vi "Two Axis Display.vi"(0 "Data In":T4 {"time" format="%<%.3X>T"}, 2 "Display State In":T2 {"Time_data" format="%<%.3X>T"}, 3 "Container State":T3) -> (6 "Data Out":T4 {"time" format="%<%.3X>T"}, 7 "Display State Out":T2 {"Time_data" format="%<%.3X>T"}, 8 "Action":T1)   [LabVIEW 2011, in "Two Axis.xctl"]
uses:
  Two Axis.xctl
  Two Axis Data.ctl
  <vilib>/_xctls/Container State.ctl
  Two Axis State.ctl
  <vilib>/_xctls/Action.ctl
  <vilib>/_xctls/XControlSupport.lvlib
panel:
  out "2_axis_Data":cluster{"Time_data":timestamp[], sgl[]}[](graph) caption="Vaisala Data"
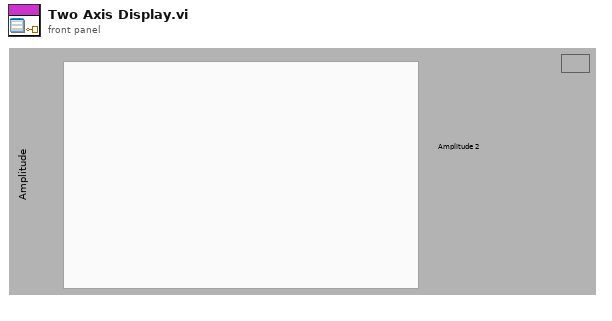
[diagram p1: front panel]
types:
  T1 = typedef "XControlSupport.lvlib/Action.ctl" = cluster{"Data Changed?":bool, "State Changed?":bool, "Action Name":string}
  T2 = typedef "Two Axis.xctl/Two Axis State.ctl" = cluster{"History":i32, "Time_data":timestamp[], "Data_Out":sgl[][], "NumPlots":i32, "LegElem":i32, "Plot Details":cluster{"Name":string, "Line Width":u8, "Line Style":u8, "Color":u32}[], "Y-Axis Labels":string[], "Title":string, "data_only?":bool}
  T3 = typedef "XControlSupport.lvlib/Container State.ctl" = cluster{"Indicator?":bool, "Run Mode?":bool, " Refnum":refnum<vi>}
  T4 = typedef "Two Axis.xctl/Two Axis Data.ctl" = cluster{"Data":sgl[], "time":timestamp}
  T5 = cluster{"Name":string, "Line Width":u8, "Line Style":u8, "Color":u32}[]
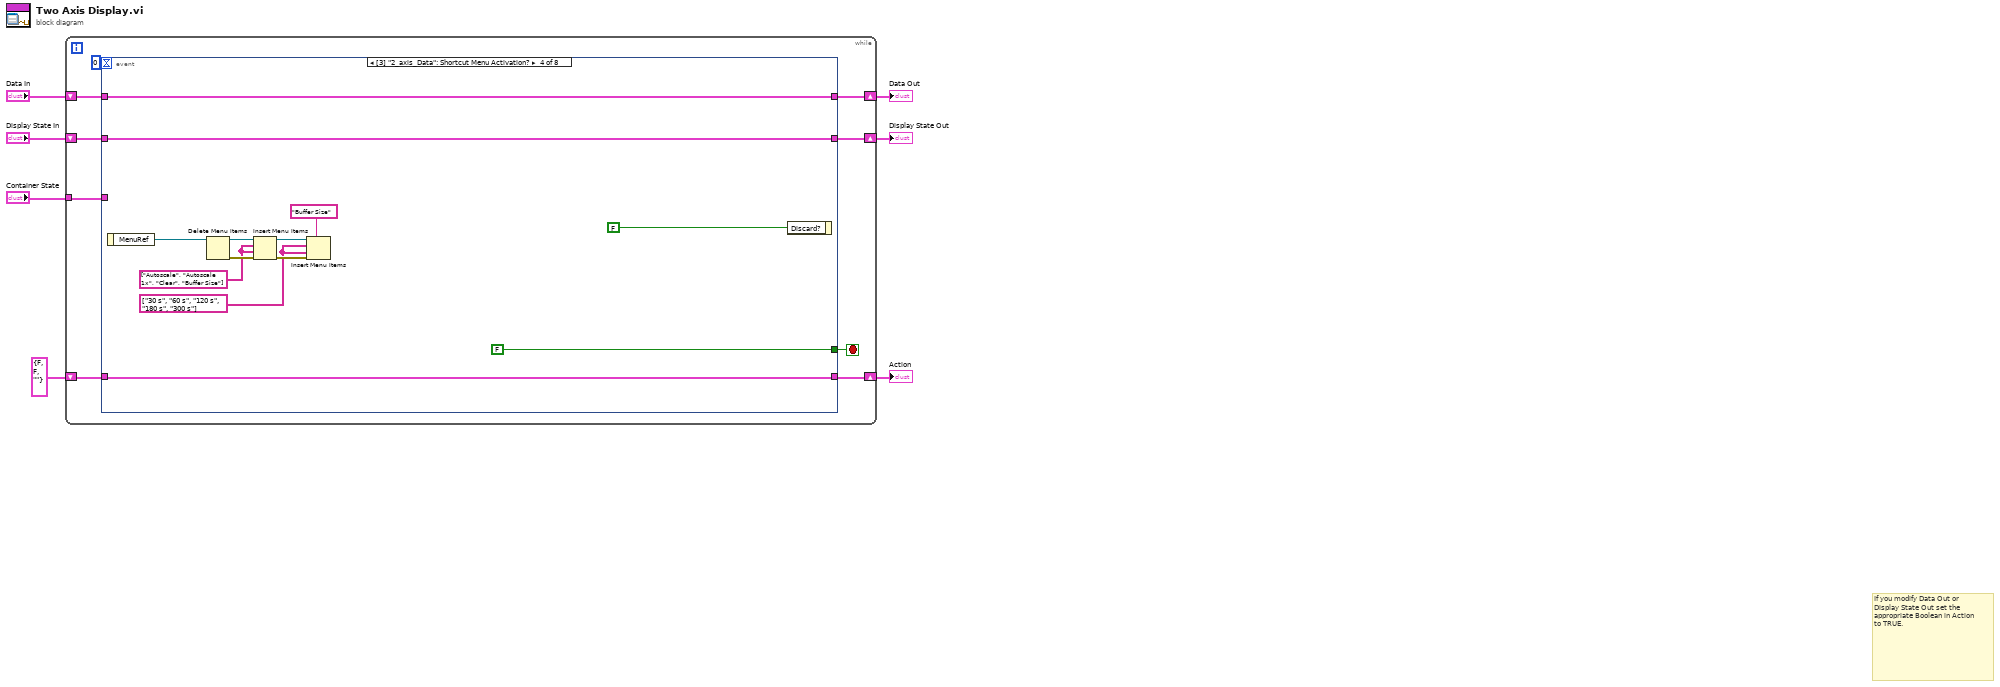
[diagram p0: block diagram]
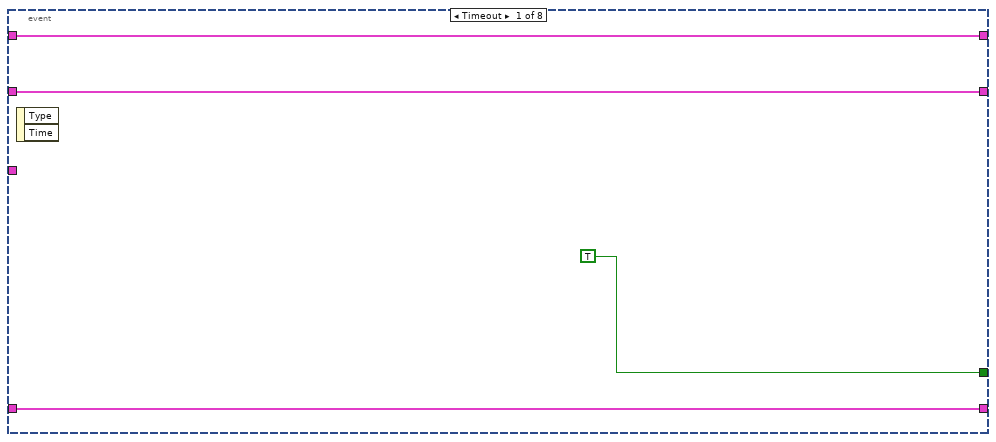
[diagram p2: hidden frame]
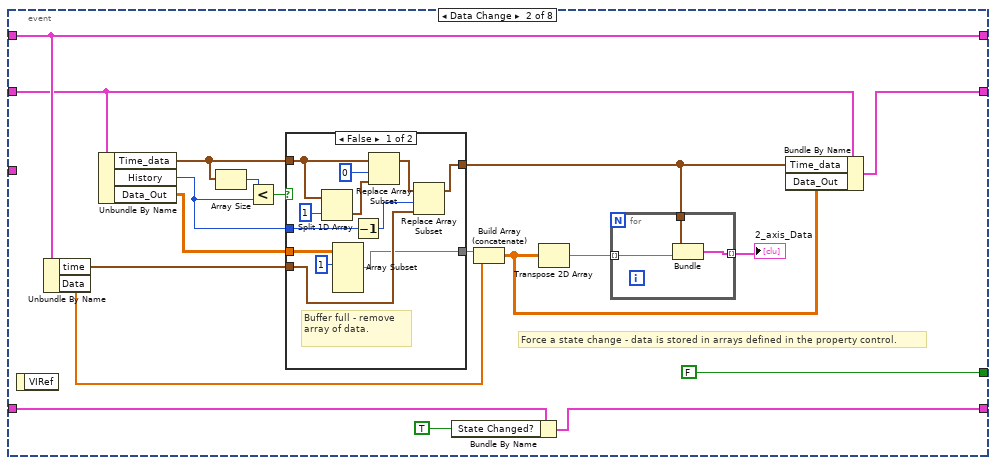
[diagram p3: hidden frame]
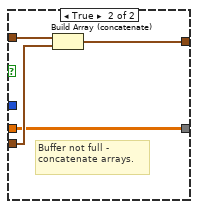
[diagram p4: hidden frame]
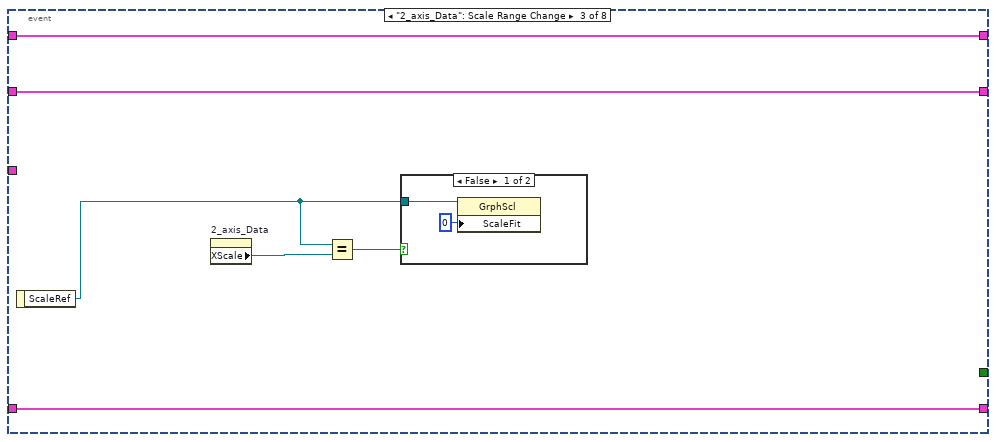
[diagram p5: hidden frame]
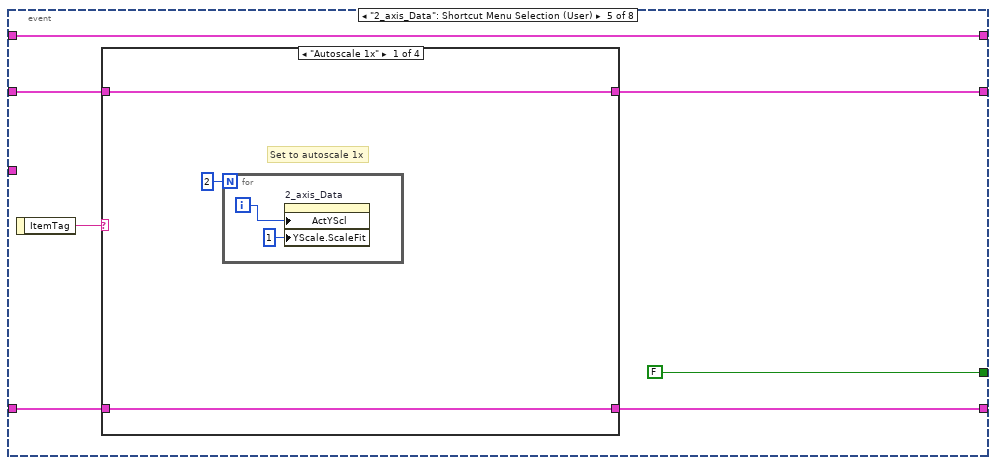
[diagram p7: hidden frame]
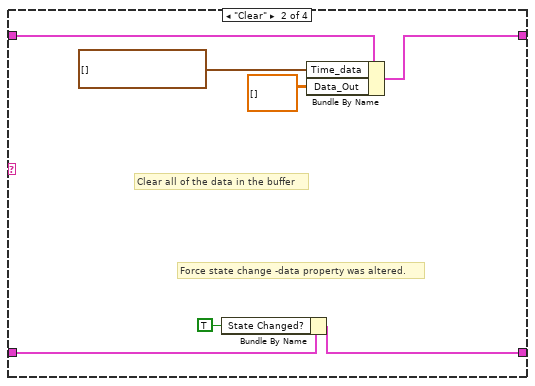
[diagram p8: hidden frame]
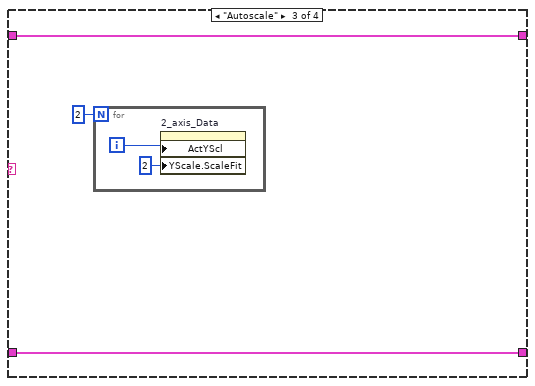
[diagram p9: hidden frame]
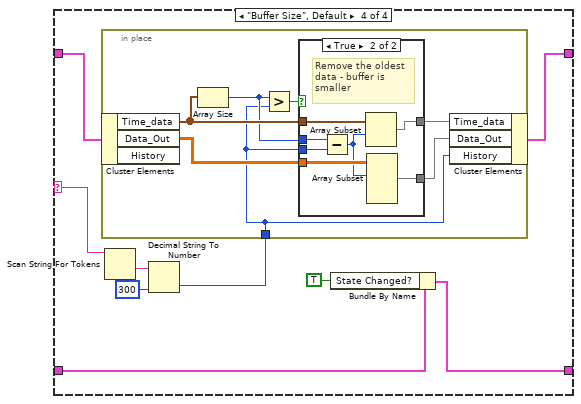
[diagram p10: hidden frame]
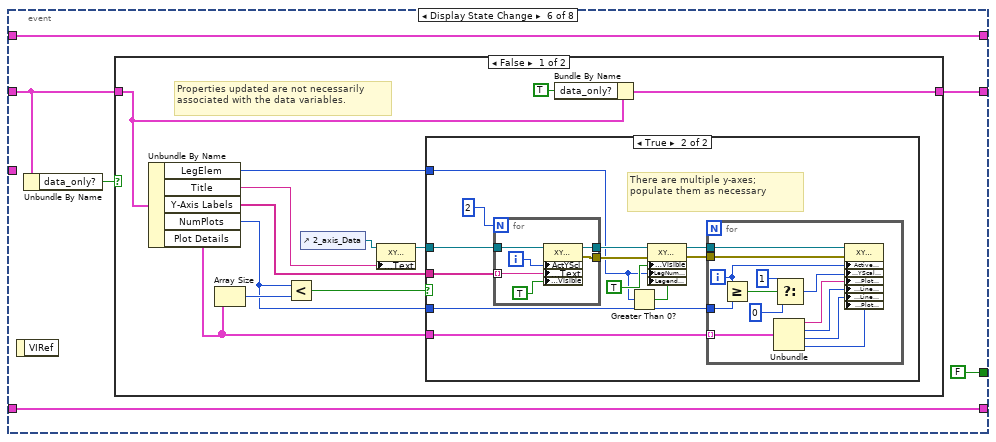
[diagram p12: hidden frame]
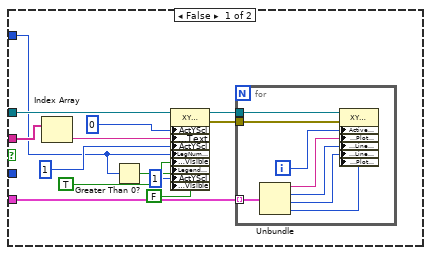
[diagram p13: hidden frame]
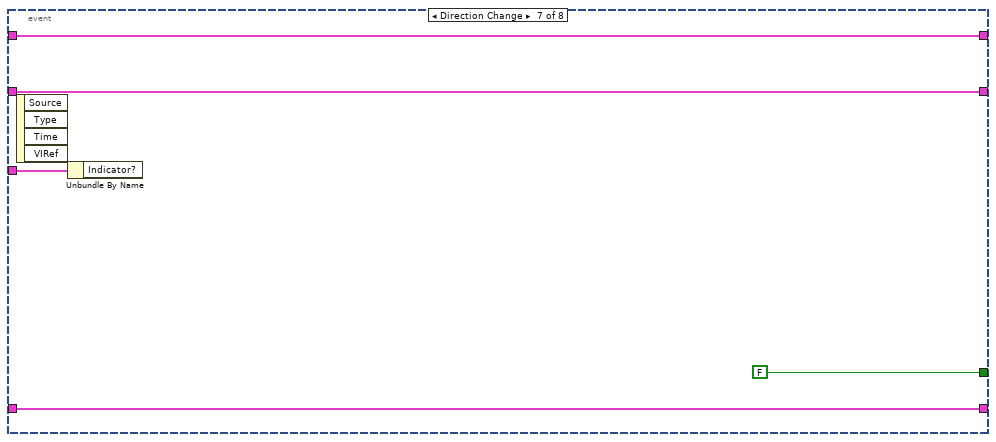
[diagram p15: hidden frame]
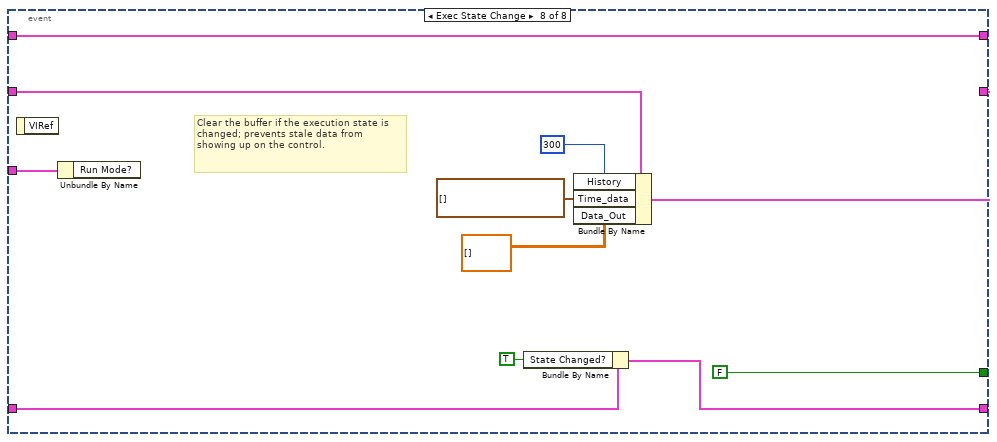
[diagram p16: hidden frame]
diagram:
  # "If you modify Data Out or\nDisplay State Out set the\nappropriate Boolean in Action\nto TRUE."
  n1 = while {
    shift-right: [w15] -> w4
    shift-left: "Display State In" -> [w16]
    tunnel: "Container State" -> [w12]
    shift-right: [w10] -> w7
    shift-left: "Data In" -> [w11]
    shift-right: [w8] -> w2
    shift-left: T1 {"Data Changed?"=FALSE, "State Changed?"=FALSE, "Action Name"=""} ("Action") -> [w9]
    stop <- w14 stop-if-true
    n2 = event shown="[3] \"2_axis_Data\": Shortcut Menu Activation?" {
      selector: _ -> [_ _ _ _ _ _ _ _]
      dyn-events: _ -> [_ _ _ _ _ _ _ _]
      timeout: 0 -> [_ _ _ _ _ _ _ _]
      tunnel: w16 -> [w18 w29 w63 w79 w84 w131 w203 w213]
      tunnel: [w18 w27 w63 w79 w82 w130 w203 w206] -> w15
      tunnel: [TRUE FALSE _ FALSE FALSE FALSE FALSE FALSE] -> w14
      tunnel: w12 -> [_ _ _ _ _ _ w204 w215]
      tunnel: w11 -> [w17 w39 w64 w78 w86 w134 w202 w214]
      tunnel: [w17 w39 w64 w78 w86 w134 w202 w214] -> w10
      tunnel: [w19 w24 w62 w77 w81 w133 w201 w207] -> w8
      tunnel: w9 -> [w19 w26 w62 w77 w83 w133 w201 w209]
      event Timeout {
        n3 = event-data() -> ()  [unwired: 1 in, 2 out]
      }
      event Data Change {
        # "Force a state change - data is stored in arrays defined in the property control."
        n4 = event-data() -> ()  [unwired: 1 in, 1 out]
        n5 = Unbundle By Name(w39) -> ("time"=w38:timestamp, "Data"=w35:sgl[])
        n6 = Unbundle By Name(w29) -> ("Time_data"=w34:timestamp[], "History"=w32:i32, "Data_Out"=w36:sgl[][])
        n7 = Array Size(array=w34) -> (size(s)=w33:i32)
        n8 = Less?(x=w33, y=w32) -> (x < y?=w31:bool)
        n9 = case shown="False" w31 {
          tunnel: w34 -> [w49 w58]
          tunnel: [w48 w56] -> w28
          tunnel: w38 -> [w47 w57]
          tunnel: w36 -> [w44 w55]
          tunnel: w32 -> [w46 _]
          tunnel: [w43 w55] -> w37
          frame False {
            # "Buffer full - remove array of data."
            n10 = Split 1D Array(array=w49, index=1) -> (second subarray=w50:timestamp[])  [unwired: 1 out]
            n11 = Array Subset(array=w44, index (row)=1 ("index")) -> (w43:sgl[][])  [unwired: 3 in]
            n12 = Decrement(x=w46) -> (x-1=w52:i32)
            n13 = Replace Array Subset(array=w49, new element=w50, index=0) -> (w53:timestamp[])
            n14 = Replace Array Subset(array=w53, new element=w47, index=w52) -> (w48:timestamp[])
          }
          frame True {
            # "Buffer not full - concatenate arrays."
            n15 = Build Array (concatenate)(w58, w57) -> (w56:timestamp[])
          }
        }
        n16 = Bundle By Name(cluster=w26, "State Changed?"=TRUE) -> (w24:T1)
        n17 = Build Array (concatenate)(w37, w35) -> (w22:sgl[][])
        n18 = Transpose 2D Array(2D array=w22) -> (transposed array=w21:sgl[][])
        n19 = for {
          tunnel: w21 -> [w40] mode=indexing
          tunnel: w28 -> [w42]
          tunnel: [w41] -> w30 mode=indexing
          n20 = Bundle("Time_data"=w42, w40) -> (w41:cluster{"Time_data":timestamp[], sgl[]})  [unwired: 1 in]
        }
        "2_axis_Data" <- w30
        n21 = Bundle By Name(cluster=w29, "Time_data"=w28, "Data_Out"=w22) -> (w27:T2)
      }
      event "2_axis_Data": Scale Range Change {
        n22 = event-data() -> ("ScaleRef"=w60:refnum<vi>)  [unwired: 1 in]
        n23 = property on="2_axis_Data" class="XYGraph (strict)"() -> ("XScale"=w61:refnum<vi>)  [unwired: 2 in, 2 out]
        n24 = Equal?(x=w60, y=w61) -> (x = y?=w59:bool)
        n25 = case shown="False" w59 {
          tunnel: w60 -> [w65 _]
          frame False {
            n26 = property class="GrphScl"(reference=w65, "ScaleFit"=u8 0 ("Scale Fit")) -> ()  [unwired: 1 in, 2 out]
          }
          frame True {
          }
        }
      }
      event "2_axis_Data": Shortcut Menu Activation? {
        w67 = string[] ["Autoscale", "Autoscale 1x", "Clear", "Buffer Size"] ("item names")
        w68 = string[] ["30 s", "60 s", "120 s", "180 s", "300 s"]
        n27 = event-data() -> ("MenuRef"=w74:refnum<k9>)  [unwired: 1 in]
        n28 = Delete Menu Items(9:w74) -> (0:w72:errorcluster, 3:w73:refnum<k9>)  [unwired: 3 in]
        n29 = Insert Menu Items(6:w72, 7:w67, 8:w67, 9:w73) -> (0:w70:errorcluster, 3:w71:refnum<k9>)  [unwired: 2 in, 1 out]
        n30 = Insert Menu Items(5:"Buffer Size", 6:w70, 7:w68, 8:w68, 9:w71) -> ()  [unwired: 1 in, 3 out]
        n31 = event-data("Discard?"=FALSE) -> ()  [unwired: 1 in, 1 out]
      }
      event "2_axis_Data": Shortcut Menu Selection (User) {
        n32 = event-data() -> ("ItemTag"=w85:string)  [unwired: 1 in]
        n33 = case shown="\"Autoscale 1x\"" w85 {
          selector: w85 -> [_ _ _ w110]
          tunnel: w84 -> [w89 w98 w101 w112]
          tunnel: w83 -> [w88 w94 w100 w106]
          tunnel: [w89 w95 w101 w111] -> w82
          tunnel: [w88 w93 w100 w104] -> w81
          frame "Autoscale 1x" {
            # "Set to autoscale 1x"
            n34 = for {
              N: 2 -> [_]
              i -> [w90]
              n35 = property on="2_axis_Data" class="XYGraph (strict)"("ActYScl"=w90, "YScale.ScaleFit"=u8 1 ("Y Scale.Scale Fit")) -> ()  [unwired: 2 in, 2 out]
            }
          }
          frame "Clear" {
            # "Force state change -data property was altered."
            # "Clear all of the data in the buffer"
            n36 = Bundle By Name(cluster=w94, "State Changed?"=TRUE) -> (w93:T1)
            n37 = Bundle By Name(cluster=w98, "Time_data"=timestamp[] [], "Data_Out"=sgl[][] []) -> (w95:T2)
          }
          frame "Autoscale" {
            n38 = for {
              N: 2 -> [_]
              i -> [w102]
              n39 = property on="2_axis_Data" class="XYGraph (strict)"("ActYScl"=w102, "YScale.ScaleFit"=u8 2 ("Y Scale.Scale Fit")) -> ()  [unwired: 2 in, 2 out]
            }
          }
          frame "Buffer Size", Default {
            n40 = Scan String For Tokens(9:w110) -> (1:w109:string)  [unwired: 5 in, 3 out]
            n41 = Decimal String To Number(string=w109, default (0L)=300 ("default (0 I32)")) -> (number=w107:i32)  [unwired: 1 in, 1 out]
            n42 = in-place {
              in-place-border: w107 -> [w113]
              n43 = in-place-cluster #1(w112) -> ("Time_data"=w118:timestamp[], "Data_Out"=w116:sgl[][])  [unwired: 1 out]
              n44 = Array Size(array=w118) -> (size(s)=w114:i32)
              n45 = Greater?(x=w114, y=w113) -> (0:w119:bool)
              n46 = case shown="True" w119 {
                tunnel: w118 -> [w121 w128]
                tunnel: [w121 w125] -> w117
                tunnel: w116 -> [w120 w124]
                tunnel: [w120 w123] -> w115
                tunnel: w114 -> [_ w127]
                tunnel: w113 -> [_ w126]
                frame False {
                  # "Buffer not filled yet or was smaller"
                }
                frame True {
                  # "Remove the oldest data - buffer is smaller"
                  n47 = Subtract(x=w127, y=w126) -> (x-y=w122:i32)
                  n48 = Array Subset(array=w128, index=w122) -> (w125:timestamp[])  [unwired: 1 in]
                  n49 = Array Subset(array=w124, index (row)=w122) -> (w123:sgl[][])  [unwired: 3 in]
                }
              }
              n50 = in-place-cluster #1("Time_data"=w117, "Data_Out"=w115, "History"=w113) -> (w111:T2)
            }
            n51 = Bundle By Name(cluster=w106, "State Changed?"=TRUE) -> (w104:T1)
          }
        }
      }
      event Display State Change {
        n52 = event-data() -> ()  [unwired: 1 in, 1 out]
        n53 = Unbundle By Name(w131) -> ("data_only?"=w132:bool)
        n54 = case shown="False" w132 {
          tunnel: w131 -> [w141 w199]
          tunnel: [w139 w199] -> w130
          frame False {
            # "Properties updated are not necessarily associated with the data variables."
            n55 = Unbundle By Name(w141) -> ("LegElem"=w142:i32, "Title"=w146:string, "Y-Axis Labels"=w135:string[], "NumPlots"=w137:i32, "Plot Details"=w136:T5)
            n56 = Array Size(array=w136) -> (size(s)=w138:i32)
            n57 = Less?(x=w137, y=w138) -> (x < y?=w144:bool)
            n58 = control-ref of="2_axis_Data"() -> (w145:refnum<vi>)
            n59 = property on="Property Node" class="XYGraph (strict)"(reference=w145, "Caption.Text"=w146) -> (reference out=w143:refnum<vi>)  [unwired: 1 in, 1 out]
            n60 = case shown="True" w144 {
              tunnel: w143 -> [w153 w178]
              tunnel: w135 -> [w158 w177]
              tunnel: w136 -> [w154 w173]
              tunnel: w137 -> [_ w172]
              tunnel: w142 -> [w150 w169]
              frame False {
                n61 = Index Array(array=w158) -> (element=w157:string)  [unwired: 1 in]
                n62 = Greater Than 0?(x=w150) -> (x > 0?=w149:bool)
                n63 = property class="XYGraph (strict)"(reference=w153, "ActYScl"=0 ("Active Y Scale"), "YScale.NameLbl.Text"=w157, "ActYScl"=1 ("Active Y Scale"), "LegNumRows"=w150, "YScale.Visible"=TRUE ("Y Scale.Visible"), "Legend Visible"=w149, "ActYScl"=1 ("Active Y Scale"), "YScale.Visible"=FALSE ("Y Scale.Visible")) -> (reference out=w155:refnum<vi>, error out=w151:errorcluster)  [unwired: 1 in]
                n64 = for {
                  tunnel: w155 -> [w167]
                  tunnel: w154 -> [w166] mode=indexing
                  tunnel: w151 -> [w160]
                  i -> [w164]
                  n65 = Unbundle(w166) -> ("Name"=w165:string, "Line Width"=w163:u8, "Line Style"=w162:u8, "Color"=w161:u32)
                  n66 = property class="XYGraph (strict)"(reference=w167, error in=w160, "Active Plot"=w164, "Plot.Plot Name"=w165, "Plot.Line Width"=w163, "Plot.Line Style"=w162, "Plot.Plot Color"=w161) -> ()  [unwired: 2 out]
                }
              }
              frame True {
                # "There are multiple y-axes; populate them as necessary"
                n67 = for {
                  N: 2 -> [_]
                  tunnel: w178 -> [w198]
                  tunnel: w177 -> [w196] mode=indexing
                  tunnel: [w195] -> w176
                  tunnel: [w193] -> w170
                  i -> [w197]
                  n68 = property class="XYGraph (strict)"(reference=w198, "ActYScl"=w197, "YScale.NameLbl.Text"=w196, "YScale.Visible"=TRUE ("Y Scale.Visible")) -> (reference out=w195:refnum<vi>, error out=w193:errorcluster)  [unwired: 1 in]
                }
                n69 = Greater Than 0?(x=w169) -> (x > 0?=w168:bool)
                n70 = property class="XYGraph (strict)"(reference=w176, error in=w170, "YScale.Visible"=TRUE ("Y Scale.Visible"), "LegNumRows"=w169, "Legend Visible"=w168) -> (reference out=w174:refnum<vi>, error out=w171:errorcluster)
                n71 = for {
                  tunnel: w174 -> [w192]
                  tunnel: w173 -> [w185] mode=indexing
                  tunnel: w172 -> [w190]
                  tunnel: w171 -> [w180]
                  i -> [w191]
                  n72 = Greater Or Equal?(x=w191, y=w190) -> (x >= y?=w189:bool)
                  n73 = Unbundle(w185) -> ("Name"=w184:string, "Line Width"=w183:u8, "Line Style"=w182:u8, "Color"=w181:u32)
                  n74 = Select(t=u32 1, s=w189, f=u32 0 ("Plot.Y Scale Index")) -> (s? t:f=w186:u32)
                  n75 = property class="XYGraph (strict)"(reference=w192, error in=w180, "Active Plot"=w191, "Plot.YScaleIdx"=w186, "Plot.Plot Name"=w184, "Plot.Line Width"=w183, "Plot.Line Style"=w182, "Plot.Plot Color"=w181) -> ()  [unwired: 2 out]
                }
              }
            }
            n76 = Bundle By Name(cluster=w141, "data_only?"=TRUE) -> (w139:T2)
          }
          frame True {
          }
        }
      }
      event Direction Change {
        n77 = event-data() -> ()  [unwired: 1 in, 4 out]
        n78 = Unbundle By Name(w204) -> ()  [unwired: 1 out]
      }
      event Exec State Change {
        # "Clear the buffer if the execution state is changed; prevents stale data from showing up on the control."
        n79 = event-data() -> ()  [unwired: 1 in, 1 out]
        n80 = Unbundle By Name(w215) -> ()  [unwired: 1 out]
        n81 = Bundle By Name(cluster=w209, "State Changed?"=TRUE) -> (w207:T1)
        n82 = Bundle By Name(cluster=w213, "History"=300, "Time_data"=timestamp[] [], "Data_Out"=sgl[][] []) -> (w206:T2)
      }
    }
  }
  "Display State Out" <- w4
  "Data Out" <- w7
  "Action" <- w2
